vi "Init Wind.vi"() -> (3 "Wind Queue Cluster":T1)   [LabVIEW 2013]
uses:
  Data/TypeDefs/WindData Queue Cluster.ctl
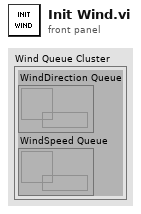
[diagram p1: front panel]
types:
  T1 = typedef "WindData Queue Cluster.ctl" = cluster{"WindDirection Queue":refnum<queue>, "WindSpeed Queue":refnum<queue>}
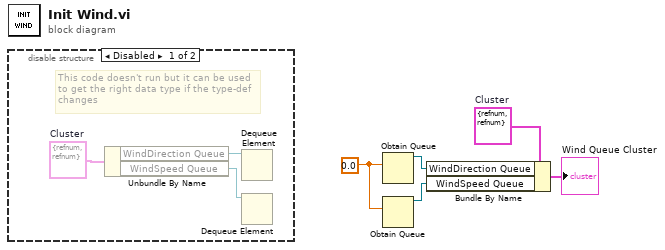
[diagram p0: block diagram]
diagram:
  w1 = 0.0 ("x")
  w5 = T1 {"WindDirection Queue"=refnum, "WindSpeed Queue"=refnum}  # Cluster
  n1 = disable-structure shown="Disabled" {
    frame Disabled {
      w6 = T1 {"WindDirection Queue"=refnum, "WindSpeed Queue"=refnum}  # Cluster
      # "This code doesn't run but it can be used to get the right data type if the type-def changes"
      n2 = Unbundle By Name(w6) -> ("WindDirection Queue"=w8:refnum<queue>, "WindSpeed Queue"=w7:refnum<queue>)
      n3 = Dequeue Element(queue=w8) -> ()  [unwired: 2 in, 4 out]
      n4 = Dequeue Element(queue=w7) -> ()  [unwired: 2 in, 4 out]
    }
    frame Enabled {
    }
  }
  n5 = Obtain Queue ("AirmarGPS-Compass Queue")(element data type=w1) -> (queue out=w4:refnum<queue>)  [unwired: 4 in, 2 out]
  n6 = Obtain Queue ("AirmarGPS-Compass Queue")(element data type=w1) -> (queue out=w3:refnum<queue>)  [unwired: 4 in, 2 out]
  n7 = Bundle By Name(cluster=w5, "WindDirection Queue"=w4, "WindSpeed Queue"=w3) -> (→"Wind Queue Cluster":T1)
